vi "read Uncertainty from txt.vi"(11 "file path":path) -> ()   [LabVIEW 2019]
uses:
  INCERTEZZA/formule.llb/Uncertainty.ctl
  INCERTEZZA/formule.llb/Global.vi
panel:
  in  "Cluster":T1
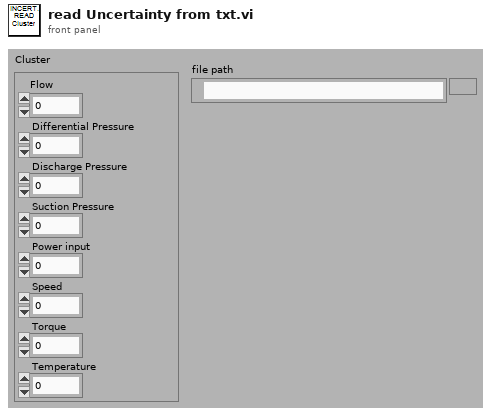
[diagram p1: front panel]
types:
  T1 = typedef "Uncertainty.ctl" = cluster{"Flow":dbl, "Differential Pressure":dbl, "Discharge Pressure":dbl, "Suction Pressure":dbl, "Power input":dbl, "Speed":dbl, "Torque":dbl, "Temperature":dbl}
  T2 = enum16{"open", "replace", "create", "open or create", "replace or create", "replace or create with confirmation"}
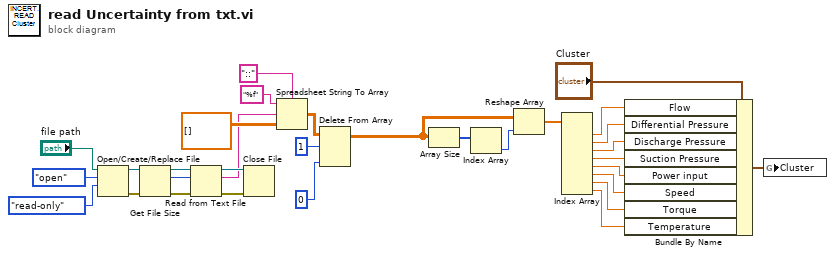
[diagram p0: block diagram]
diagram:
  n1 = Open/Create/Replace File(file path (use dialog)="file path", operation (0:open)=T2."open", access (0:read/write)=enum16{"read/write", "read-only", "write-only"}."read-only") -> (refnum out=w27:refnum<file>, error out=w28:errorcluster)  [unwired: 1 in, 3 out]
  n2 = Get File Size(file=w27, error in=w28) -> (refnum out=w26:refnum<file>, size (in bytes)=w25:i64, 0:w24:errorcluster)
  n3 = Read from Text File(file (use dialog)=w26, count=w25, error in=w24) -> (refnum out=w31:refnum<file>, text=w13:string, error out=w30:errorcluster)  [unwired: 2 out]
  n4 = Close File(refnum=w31, error in=w30) -> ()  [unwired: 2 out]
  n5 = Spreadsheet String To Array(delimiter (Tab)="::", format string="%f", spreadsheet string=w13, array type (2D Dbl)=dbl[][] [] ("Array")) -> (array=w20:dbl[][])
  n6 = Delete From Array "Delete From Array"(array=w20, length=1, index (col)=0 ("disabled index (col)")) -> (array with subset deleted=w16:dbl[][])  [unwired: 1 in, 1 out]
  n7 = Array Size(array=w16) -> (size(s)=w15:i32[])
  n8 = Index Array(array=w15) -> (element=w14:i32)  [unwired: 1 in]
  n9 = Reshape Array(w16, w14) -> (w12:dbl[])
  n10 = Index Array(array=w12) -> (element #1=w9:dbl, element #2=w8:dbl, element #3=w7:dbl, element #4=w6:dbl, element #5=w5:dbl, element #6=w4:dbl, element #7=w3:dbl, element #8=w2:dbl)  [unwired: 8 in]
  n11 = Bundle By Name(cluster="Cluster", "Flow"=w9, "Differential Pressure"=w8, "Discharge Pressure"=w7, "Suction Pressure"=w6, "Power input"=w5, "Speed"=w4, "Torque"=w3, "Temperature"=w2) -> (w10:T1)
  n12 = global write "Global.vi" "Cluster"(w10) -> ()
